vi "get_FPGA_VI_ref.vi"(8 "error in (no error)":errorcluster, 11 "FPGAWrapperAN110607Galvo in":refnum<class "FPGAWrapperAN110607Galvo.lvclass">) -> (0 "error out":errorcluster, 2 "FPGA VI reference":T1, 3 "FPGAWrapperAN110607Galvo out":refnum<class "FPGAWrapperAN110607Galvo.lvclass">)   [LabVIEW 2010, in "FPGAWrapperAN110607Galvo.lvclass"]
uses:
  FPGAWrapperAN110607Galvo.lvclass
  FPGA_VI_ref.ctl
  class_data.vi
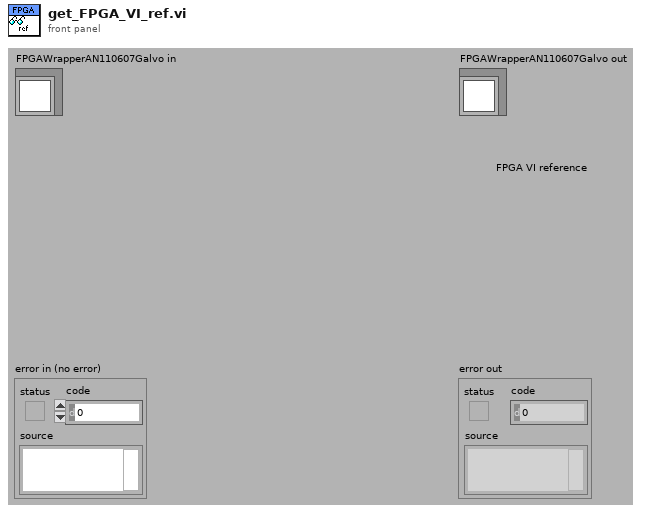
[diagram p1: front panel]
types:
  T1 = typedef "FPGAWrapperAN110607Galvo.lvclass/FPGA_VI_ref.ctl" = refnum<k20>
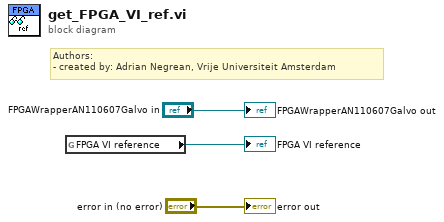
[diagram p0: block diagram]
diagram:
  # "Authors: \n- created by: Adrian Negrean, Vrije Universiteit Amsterdam"
  n1 = global read "class_data.vi" "FPGA VI reference"() -> (→"FPGA VI reference":T1)
  "error out" <- "error in (no error)"
  "FPGAWrapperAN110607Galvo out" <- "FPGAWrapperAN110607Galvo in"
